vi "ModifyGraph axThick.vi"(8 "error in (no error)":errorcluster, 10 "Axes Thickness (points)":T1, 11 "ITX Commands in":refnum<class "ITX Commands.lvclass">) -> (0 "error out":errorcluster, 3 "ITX Commands out":refnum<class "ITX Commands.lvclass">)   [LabVIEW 2020, in "ITX Commands.lvclass"]
uses:
  ITX Commands.lvclass
panel:
  out "resulting string":string
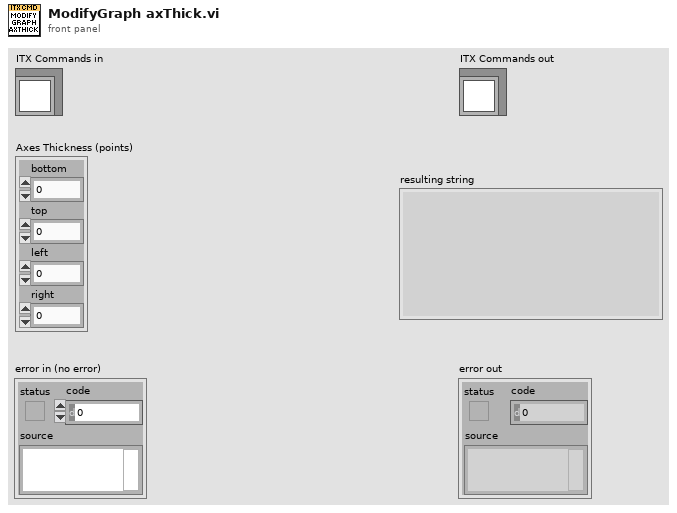
[diagram p1: front panel]
types:
  T1 = cluster{"bottom":dbl, "top":dbl, "left":dbl, "right":dbl}
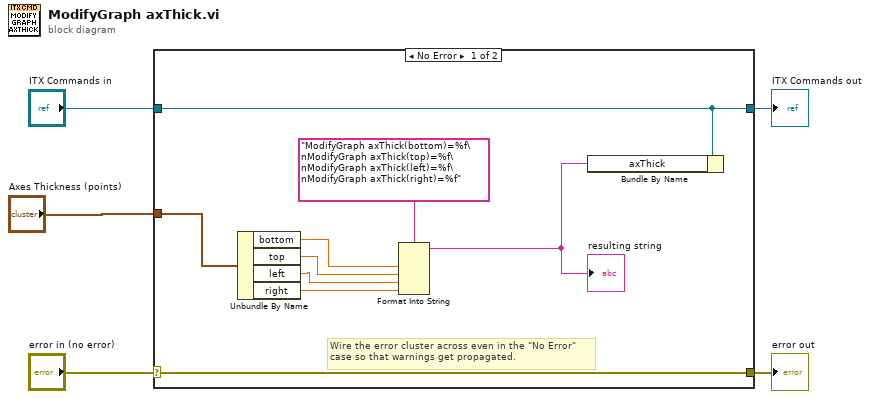
[diagram p0: block diagram]
diagram:
  n1 = case shown="No Error" "error in (no error)" {
    selector: "error in (no error)" -> [w14 w16]
    tunnel: [w14 w16] -> w4
    tunnel: [w7 w15] -> w2
    tunnel: "ITX Commands in" -> [w7 w15]
    tunnel: "Axes Thickness (points)" -> [w13 _]
    frame No Error {
      # "Wire the error cluster across even in the \"No Error\"\ncase so that warnings get propagated."
      n2 = Unbundle By Name(w13) -> ("bottom"=w9:dbl, "top"=w10:dbl, "left"=w11:dbl, "right"=w12:dbl)
      n3 = Format Into String(format string="ModifyGraph axThick(bottom)=%f\nModifyGraph axThick(top)=%f\nModifyGraph axThick(left)=%f\nModifyGraph axThick(right)=%f", w9, w10, w11, w12) -> (resulting string=w6:string)  [unwired: 2 in, 1 out]
      "resulting string" <- w6
      n4 = Bundle By Name(cluster=w7, "axThick"=w6) -> ()  [unwired: 1 out]
    }
    frame Error {
    }
  }
  "error out" <- w4
  "ITX Commands out" <- w2
